vi "Phase_curv.vi"() -> ()   [LabVIEW 2013]
uses:
  <vilib>/ptbypt/NI_PtbyPt.lvlib
panel:
  in  "Имя файла 2":path=path "pha(w).xlsx"
  in  "alphas":dbl[](array[numeric])
  in  "Имя файла":path=path "pha(w).xlsx"
  in  "samples  per chip":i32=2
  in  "chips per symb":i32=64
  in  "symb_rate(Hz)":dbl=2500000.0
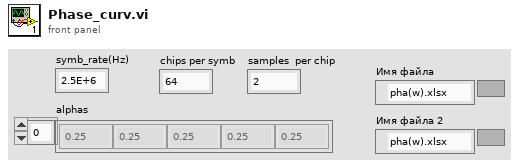
[diagram p1: front panel]
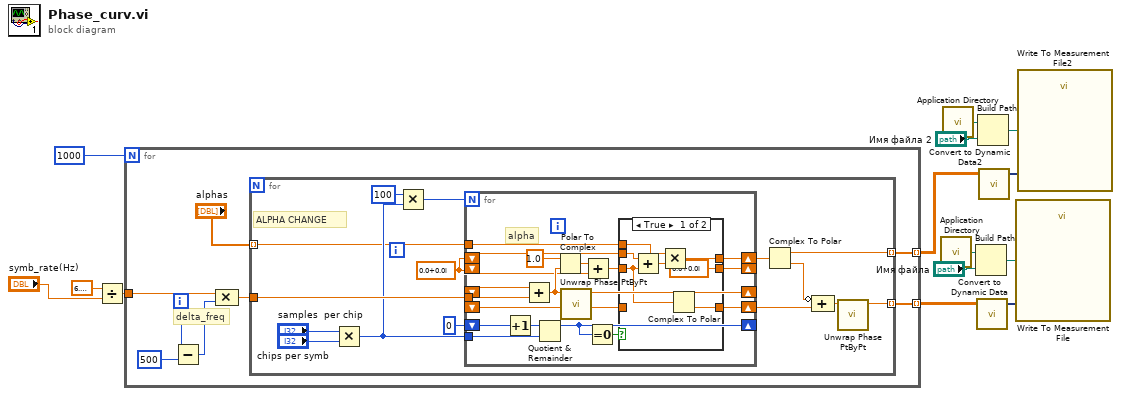
[diagram p0: block diagram]
diagram:
  n1 = Divide(x=6.283185307179586, y="symb_rate(Hz)") -> (x/y=w12:dbl)
  n2 = for {
    N: 1000 -> [_]
    tunnel: [w20] -> w6 mode=indexing
    tunnel: w12 -> [w21]
    tunnel: [w15] -> w1 mode=indexing
    i -> [w19]
    # "delta_freq"
    n3 = Subtract(x=w19, y=500) -> (x-y=w18:i32)
    n4 = Compound Arithmetic op=MULTIPLY(w21, w18) -> (w22:dbl)
    n5 = for {
      tunnel: w22 -> [w31]
      tunnel: [w26] -> w20 mode=indexing
      tunnel: "alphas" -> [w24] mode=indexing
      tunnel: [w23] -> w15 mode=indexing
      w27 = cdb 0.0+0.0i
      # "ALPHA CHANGE"
      n6 = Multiply(x="samples  per chip", y="chips per symb") -> (x*y=w29:i32)
      n7 = Multiply(x=100, y=w29) -> (x*y=w30:i32)
      n8 = for {
        N: w30 -> [_]
        shift-right: [w56] -> _
        shift-left: _ -> [w55]
        shift-right: [w38] -> _
        shift-left: 0 -> [w50]
        shift-right: [w48] -> _
        shift-left: w27 -> [w47]
        shift-right: [w46] -> w32
        shift-left: w27 -> [w45]
        shift-right: [w44] -> w34
        shift-left: _ -> [w42]
        tunnel: w31 -> [w43]
        tunnel: w29 -> [w41]
        tunnel: w24 -> [w40]
        # "alpha"
        n9 = Increment(x=w50) -> (x+1=w51:i32)
        n10 = Add(x=w55, y=w43) -> (x+y=w54:dbl)
        n11 = Quotient & Remainder(x=w51, y=w41) -> (x-y*floor(x/y)=w38:i32)  [unwired: 1 out]
        n12 = Polar To Complex(1:w54, 2:1.0 ("r")) -> (0:w52:cdb)
        n13 = call <vilib>:"Unwrap Phase PtByPt.vi"("phase"=w54) -> ("unwrapped phase"=w56:dbl)  [unwired: 10 in]
        n14 = Add(x=w52, y=w47) -> (x+y=w49:cdb)
        n15 = Equal To 0?(x=w38) -> (x = 0?=w39:bool)
        n16 = case shown="True" w39 {
          tunnel: w49 -> [w60 w66]
          tunnel: [cdb 0.0+0.0i w66] -> w48
          tunnel: [w61 w65] -> w46
          tunnel: w45 -> [w59 w65]
          tunnel: [w58 w64] -> w44
          tunnel: w42 -> [_ w64]
          tunnel: w40 -> [w57 _]
          frame True {
            n17 = Add(x=w59, y=w60) -> (x+y=w62:cdb)
            n18 = Multiply(x=w57, y=w62) -> (x*y=w61:cdb)
            n19 = Complex To Polar(r * e^(i*theta)=w60) -> (theta=w58:dbl)  [unwired: 1 out]
          }
          frame False {
          }
        }
      }
      n20 = Complex To Polar(r * e^(i*theta)=w32) -> (r=w23:dbl, theta=w33:dbl)
      n21 = Compound Arithmetic op=ADD(invert w33, w34) -> (w25:dbl)
      n22 = call <vilib>:"Unwrap Phase PtByPt.vi"("phase"=w25) -> ("unwrapped phase"=w26:dbl)  [unwired: 10 in]
    }
  }
  n23 = call <vilib>:"Application Directory.vi"() -> ("Application Directory"=w10:path)
  n24 = call <vilib>:"Application Directory.vi"() -> ("Application Directory"=w5:path)
  n25 = Build Path(base path=w10, name or relative path="Имя файла") -> (appended path=w8:path)
  n26 = call "Convert to Dynamic Data"("2D Array"=w6) -> ("Dynamic Data Type"=w9:dynamicdata)  [unwired: 3 in]
  n27 = Build Path(base path=w5, name or relative path="Имя файла 2") -> (appended path=w3:path)
  n28 = call "Convert to Dynamic Data2"("2D Array"=w1) -> ("Dynamic Data Type"=w4:dynamicdata)  [unwired: 3 in]
  n29 = call "Write To Measurement File"("Signals"=w9, "Filename"=w8) -> ()  [unwired: 15 in, 3 out]
  n30 = call "Write To Measurement File2"("Signals"=w4, "Filename"=w3) -> ()  [unwired: 15 in, 3 out]
